vi "Write_parameter.vi"(8 "error in (no error)":errorcluster caption="entrée d'erreur (pas d'erreur)", 10 "Parameter":string, 11 "Class Instrument Patterm_Matching en entrée":refnum<class "Class Instrument Patterm_Matching.lvclass">) -> (0 "error out":errorcluster caption="sortie d'erreur", 3 "Class Instrument Patterm_Matching en sortie":refnum<class "Class Instrument Patterm_Matching.lvclass">)   [LabVIEW 2020, in "Library Instrument & Equipement.lvlib" / "Library Instruments.lvlib" / "Class Instrument Patterm_Matching.lvclass"]
uses:
  Class Instrument Patterm_Matching.lvclass
  Commun VI/TypeDef/Commande Pattern_Matching/Commande Parameter.ctl
  Camera/Class Camera Pattern Matching (Default)/Class Pattern Matching (Default).lvclass
  JSON API/JSON Value/Set from JSON string.vi
  Instrument (Default)/Class Instrument (Default).lvclass
  JSON API/JSON Value/JSON Value.lvclass
  Class Instrument Patterm_Matching.lvclass/Class Instrument Patterm_Matching.ctl
  JSON API/Variant JSON/Variant JSON.lvlib
  JSON API/Get Polymorphic/JSON GetSet.lvlib
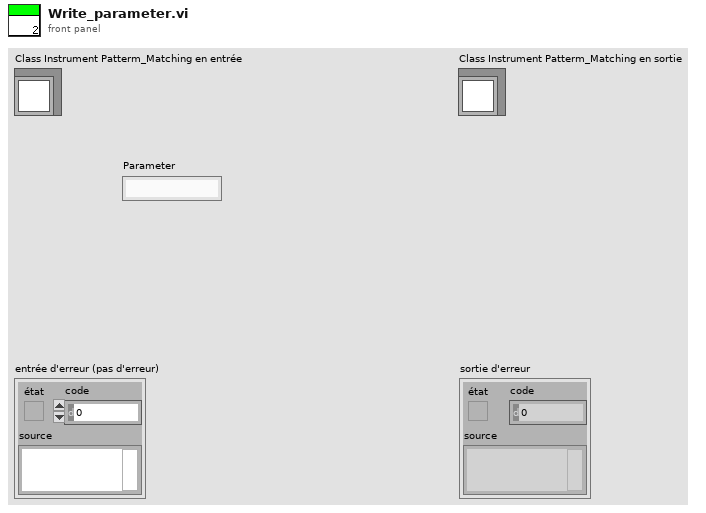
[diagram p1: front panel]
types:
  T1 = typedef "Commande Parameter.ctl" = cluster{"Device_Addr":string, "Port":string, "Number Prog":string, "Test Number":u16, "Timeout":u16, "Library Pattern Matching":refnum<class "Class Pattern Matching (Default).lvclass">}
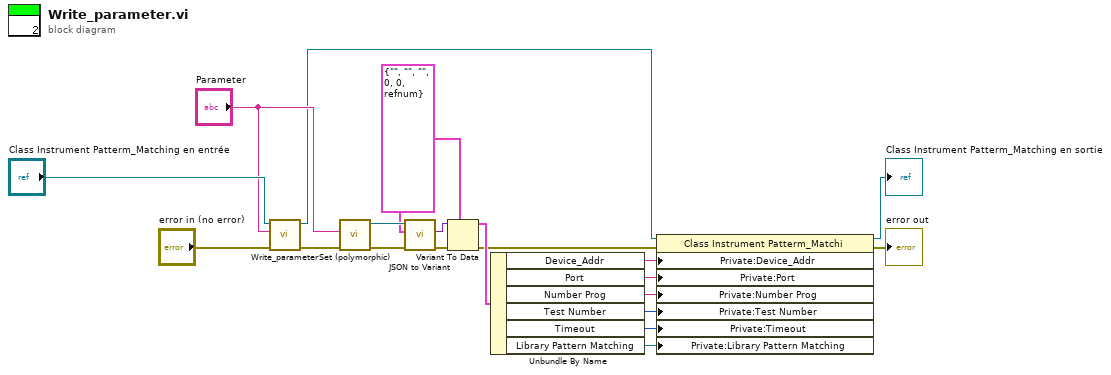
[diagram p0: block diagram]
diagram:
  w8 = T1 {"Device_Addr"="", "Port"="", "Number Prog"="", "Test Number"=0, "Timeout"=0, "Library Pattern Matching"=refnum} ("Parameter")
  n1 = call-parent "Write_parameter.vi"("error in (no error)"="error in (no error)", "Parameter"="Parameter", "Class Instrument (Default) en entrée"="Class Instrument Patterm_Matching en entrée") -> ("error out"=w15:errorcluster, "Class Instrument (Default) en sortie"=w12:refnum<class "Class Instrument Patterm_Matching.lvclass">)  [unwired: 7 in]
  n2 = call-poly "Set (polymorphic).vi"("error in (no error)"=w15, "JSON stream"="Parameter") -> ("error out"=w18:errorcluster, "JSON Value out"=w20:refnum<class "JSON Value.lvclass">)  [unwired: 7 in, 1 out]
  n3 = call "JSON to Variant.vi"("error in (no error)"=w18, "Variant (Data Type)"=w8, "JSON Value"=w20) -> ("error out"=w19:errorcluster, "Variant out"=w17:variant)  [unwired: 7 in]
  n4 = Variant To Data(error in=w19, type=w8, Variant=w17) -> (data=w16:T1, error out=w2:errorcluster)
  n5 = Unbundle By Name(w16) -> ("Device_Addr"=w7:string, "Port"=w6:string, "Number Prog"=w5:string, "Test Number"=w4:u16, "Timeout"=w3:u16, "Library Pattern Matching"=w1:refnum<class "Class Pattern Matching (Default).lvclass">)
  n6 = property class="Class Instrument Patterm_Matchi"(reference=w12, error in=w2, "Private:Device_Addr"=w7, "Private:Port"=w6, "Private:Number Prog"=w5, "Private:Test Number"=w4, "Private:Timeout"=w3, "Private:Library Pattern Matching"=w1) -> (reference out=→"Class Instrument Patterm_Matching en sortie":refnum<class "Class Instrument Patterm_Matching.lvclass">, error out=→"error out":errorcluster)
